vi "QM_Set Cursor.vi"(8 "error in (no error)":errorcluster, 10 "L":dbl, 11 "XYGraph in":refnum<vi>) -> (0 "error out":errorcluster)   [LabVIEW 2023]
doc: "Set the cursor positions on the Wave Function or Probability Density graph."
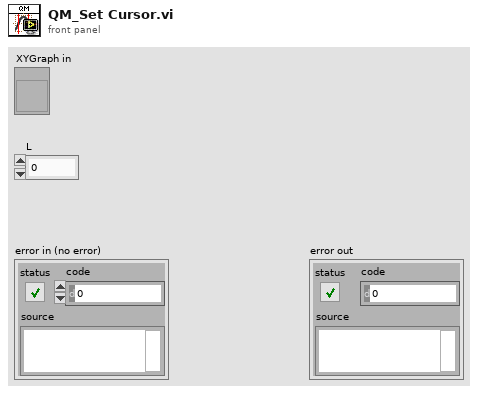
[diagram p1: front panel]
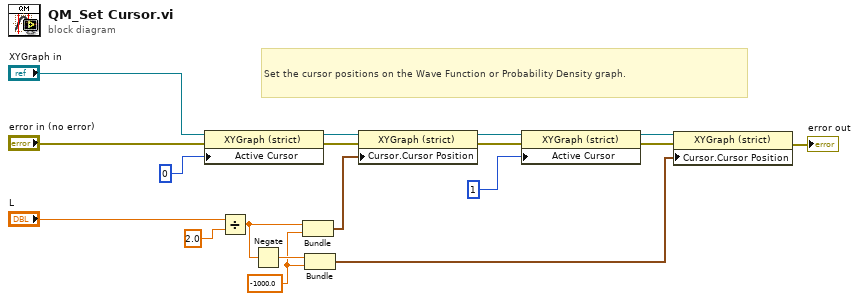
[diagram p0: block diagram]
diagram:
  w15 = -1000.0 ("y")
  # "Set the cursor positions on the Wave Function or Probability Density graph."
  n1 = property class="XYGraph (strict)"(reference="XYGraph in", error in="error in (no error)", "Active Cursor"=u32 0) -> (reference out=w8:refnum<vi>, error out=w9:errorcluster)
  n2 = Divide(x="L", y=2.0) -> (x/y=w16:dbl)
  n3 = Negate(x=w16) -> (-x=w17:dbl)
  n4 = Bundle(w16, "y"=w15) -> (w11:cluster{dbl, "y":dbl})  [unwired: 1 in]
  n5 = Bundle(w17, "y"=w15) -> (w18:cluster{dbl, "y":dbl})  [unwired: 1 in]
  n6 = property class="XYGraph (strict)"(reference=w8, error in=w9, "Cursor.Cursor Position"=w11) -> (reference out=w12:refnum<vi>, error out=w4:errorcluster)
  n7 = property class="XYGraph (strict)"(reference=w12, error in=w4, "Active Cursor"=u32 1) -> (reference out=w14:refnum<vi>, error out=w3:errorcluster)
  n8 = property class="XYGraph (strict)"(reference=w14, error in=w3, "Cursor.Cursor Position"=w18) -> (error out=→"error out":errorcluster)  [unwired: 1 out]
